vi "rampa.vi"(6 "tempo ciclo (ms)":u32, 7 "Valore massimo":dbl=50.0 format="%#_13g", 8 "Tempo di stabilizzazione (s)":dbl=5.0, 9 "reale":dbl, 10 "set":dbl, 11 "tempo rampa (s)":dbl) -> (0 "fine rampa":bool, 1 "OUT":dbl)   [LabVIEW 2019]
panel:
  # "Rampa di durata \"Tempo rampa (s)\"\nda 0 a \"Valore Massimo\""
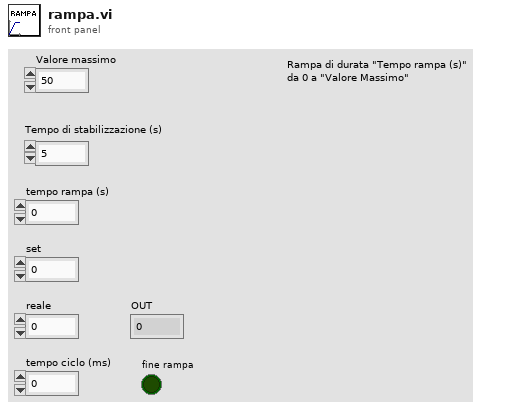
[diagram p1: front panel]
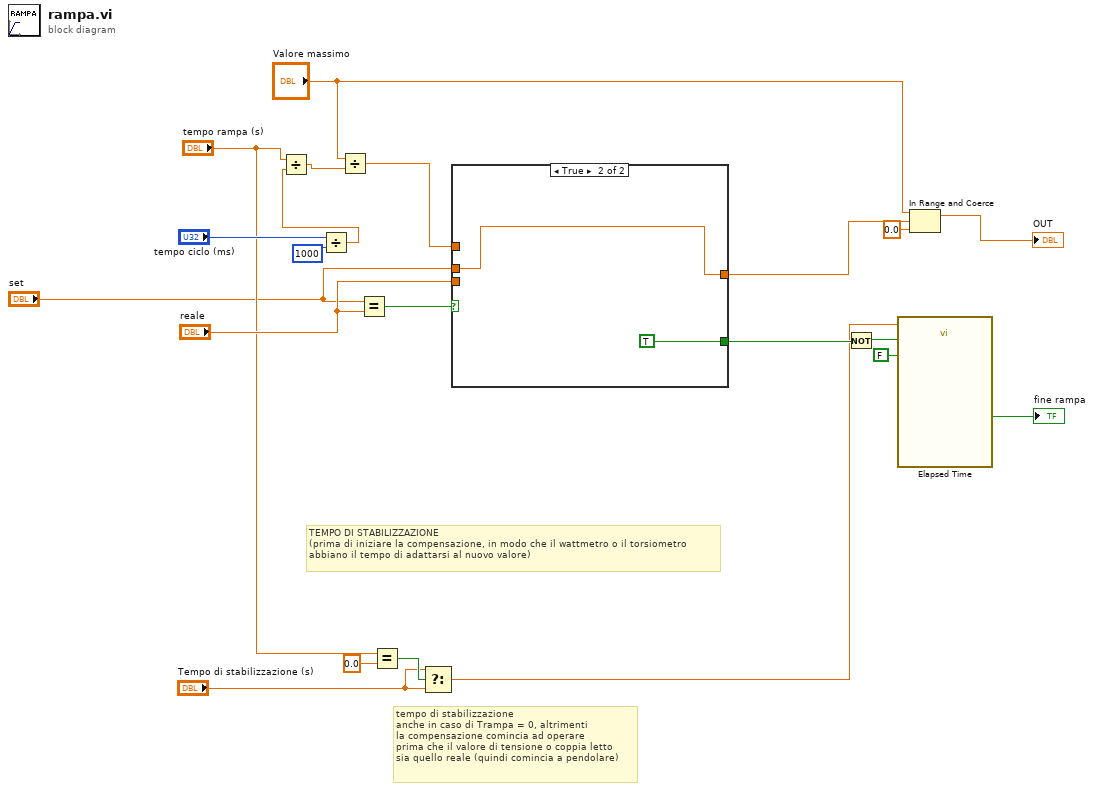
[diagram p0: block diagram]
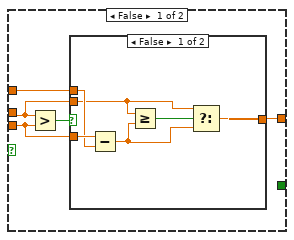
[diagram p2: hidden frame]
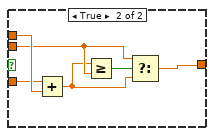
[diagram p3: hidden frame]
diagram:
  # "tempo di stabilizzazione\nanche in caso di Trampa = 0, altrimenti\nla compensazione comincia ad operare \nprima che il valore di tensione o coppia letto\nsia quello reale (quindi comincia a pendolare)"
  # "TEMPO DI STABILIZZAZIONE \n(prima di iniziare la compensazione, in modo che il wattmetro o il torsiometro\nabbiano il tempo di adattarsi al nuovo valore)"
  n1 = Divide(x="tempo ciclo (ms)", y=u32 1000) -> (x/y=w21:dbl)
  n2 = Divide(x="tempo rampa (s)", y=w21) -> (x/y=w17:dbl)
  n3 = Divide(x="Valore massimo", y=w17) -> (x/y=w18:dbl)
  n4 = Equal?(x="set", y="reale") -> (x = y?=w15:bool)
  n5 = Equal?(x="tempo rampa (s)", y=0.0) -> (x = y?=w8:bool)
  n6 = Select(t="Tempo di stabilizzazione (s)", s=w8, f="Tempo di stabilizzazione (s)") -> (s? t:f=w7:dbl)
  n7 = case shown="True" w15 {
    tunnel: "set" -> [w22 w40]
    tunnel: [w23 w40] -> w4
    tunnel: "reale" -> [w25 _]
    tunnel: w18 -> [w24 _]
    tunnel: [_ TRUE ("fine rampa")] -> w11
    frame False {
      n8 = Greater?(x=w22, y=w25) -> (0:w26:bool)
      n9 = case shown="False" w26 {
        tunnel: w25 -> [w32 w37]
        tunnel: w24 -> [w31 w38]
        tunnel: [w28 w33] -> w23
        tunnel: w22 -> [w30 w36]
        frame False {
          n10 = Subtract(x=w32, y=w31) -> (x-y=w29:dbl)
          n11 = Greater Or Equal?(x=w30, y=w29) -> (x >= y?=w27:bool)
          n12 = Select(t=w30, s=w27, f=w29) -> (s? t:f=w28:dbl)
        }
        frame True {
          n13 = Add(x=w37, y=w38) -> (x+y=w35:dbl)
          n14 = Greater Or Equal?(x=w35, y=w36) -> (x >= y?=w34:bool)
          n15 = Select(t=w36, s=w34, f=w35) -> (s? t:f=w33:dbl)
        }
      }
    }
    frame True {
    }
  }
  n16 = Not(x=w11) -> (.not. x?=w13:bool)
  n17 = call "Elapsed Time"("Time Target (s)"=w7, "Reset"=w13, "Auto Reset"=FALSE) -> ("Time has Elapsed"=→"fine rampa":bool)  [unwired: 9 in, 7 out]
  n18 = In Range and Coerce(upper limit="Valore massimo", x=w4, lower limit=0.0) -> (coerced(x)=→"OUT":dbl)  [unwired: 1 out]
